vi "subParseForComponents.vi"(8 "error in (no error)":errorcluster, 9 "Parent layer":string, 10 "Parent component":string, 11 "Refnum in":refnum<k20>) -> (0 "error out":errorcluster, 1 "Rules":T1(array[cluster]), 3 "Refnum out":refnum<k20>)   [LabVIEW 2020, in "DefaultExtensions.lvlib" / "CDefaultRuleFileParser.lvclass"]
uses:
  CDefaultRuleFileParser.lvclass
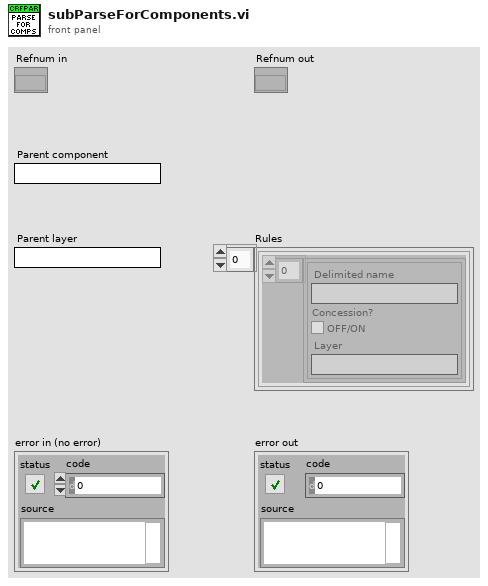
[diagram p1: front panel]
types:
  T1 = cluster{cluster{"Delimited name":string, "Concession?":bool, "Layer":string}[]}[]
  T2 = cluster{"Delimited name":string, "Concession?":bool, "Layer":string}
  T3 = cluster{"Delimited name":string, "Concession?":bool, "Layer":string}[]
  T4 = cluster{cluster{"Delimited name":string, "Concession?":bool, "Layer":string}[]}
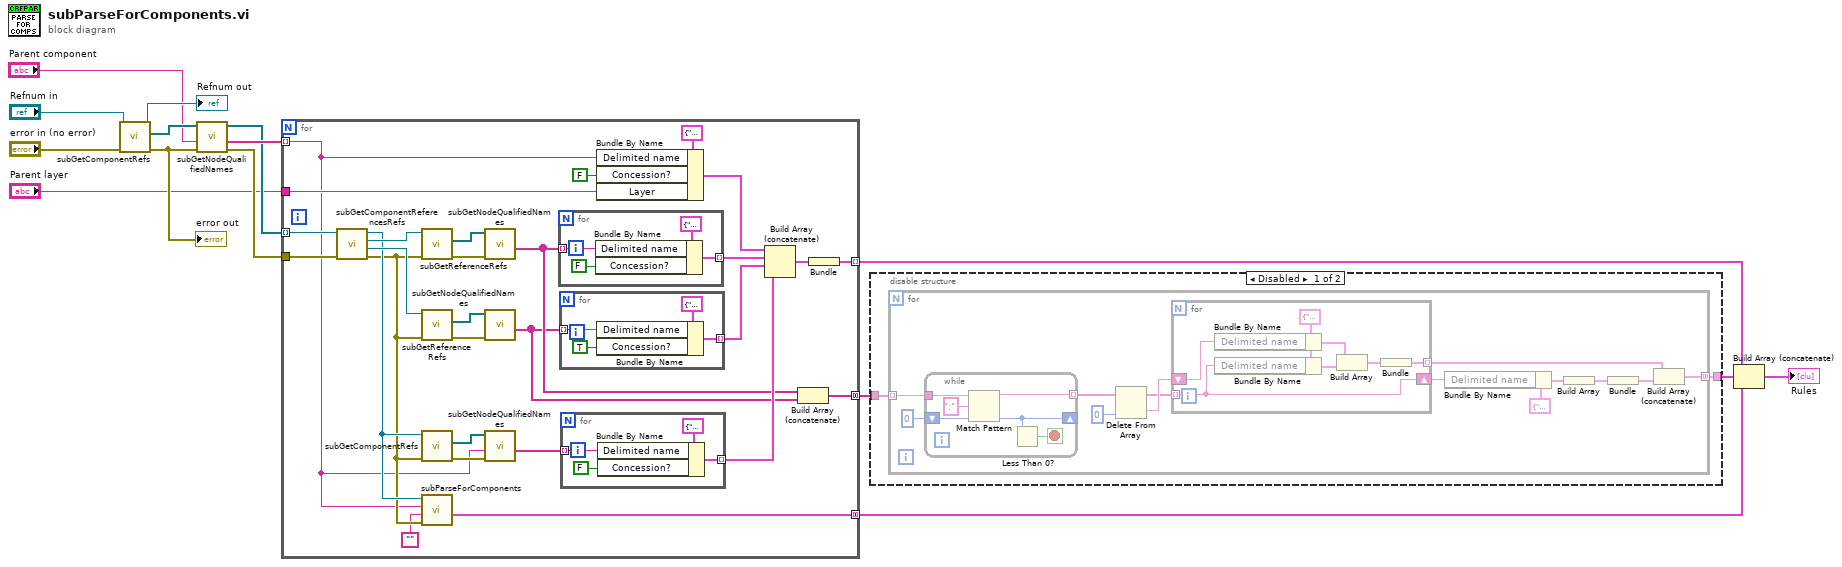
[diagram p0: block diagram]
diagram:
  n1 = call "subGetComponentRefs.vi"("error in (no error)"="error in (no error)", "Refnum in"="Refnum in") -> ("error out"=w15:errorcluster, "node result array"=w13:refnum<k20>[], "Refnum out"=→"Refnum out":refnum<k20>)  [unwired: 7 in]
  "error out" <- w15
  n2 = call "subGetNodeQualifiedNames.vi"("error in (no error)"=w15, "Parent node"="Parent component", "node[] in"=w13) -> ("error out"=w10:errorcluster, "node name[]"=w11:string[], "node[]"=w9:refnum<k20>[])  [unwired: 6 in]
  n3 = for {
    tunnel: w11 -> [w20] mode=indexing
    tunnel: [w34] -> w7 mode=indexing
    tunnel: w10 -> [w33]
    tunnel: w9 -> [w32] mode=indexing
    tunnel: "Parent layer" -> [w23]
    tunnel: [w28] -> w5 mode=concatenating
    tunnel: [w16] -> w1 mode=concatenating
    n4 = call "subGetComponentReferencesRefs.vi"("error in (no error)"=w33, "Refnum in"=w32) -> ("error out"=w24:errorcluster, "Concession Node Ref out"=w42:refnum<k20>, "Allow Node Ref out"=w43:refnum<k20>, "Refnum out"=w25:refnum<k20>)  [unwired: 6 in]
    n5 = call "subGetReferenceRefs.vi"("error in (no error)"=w24, "Refnum in"=w43) -> ("error out"=w40:errorcluster, "node result array"=w41:refnum<k20>[])  [unwired: 7 in, 1 out]
    n6 = call "subGetReferenceRefs.vi"("error in (no error)"=w24, "Refnum in"=w42) -> ("error out"=w38:errorcluster, "node result array"=w39:refnum<k20>[])  [unwired: 7 in, 1 out]
    n7 = call "subGetComponentRefs.vi"("error in (no error)"=w24, "Refnum in"=w25) -> ("error out"=w27:errorcluster, "node result array"=w26:refnum<k20>[])  [unwired: 7 in, 1 out]
    n8 = call "subParseForComponents.vi"("error in (no error)"=w24, "Parent layer"="", "Parent component"=w20, "Refnum in"=w25) -> ("Rules"=w28:T1)  [unwired: 5 in, 2 out]
    n9 = call "subGetNodeQualifiedNames.vi"("error in (no error)"=w40, "node[] in"=w41) -> ("node name[]"=w18:string[])  [unwired: 7 in, 2 out]
    n10 = call "subGetNodeQualifiedNames.vi"("error in (no error)"=w38, "node[] in"=w39) -> ("node name[]"=w17:string[])  [unwired: 7 in, 2 out]
    n11 = call "subGetNodeQualifiedNames.vi"("error in (no error)"=w27, "Parent node"=w20, "node[] in"=w26) -> ("node name[]"=w22:string[])  [unwired: 6 in, 2 out]
    n12 = for {
      tunnel: w18 -> [w54] mode=indexing
      tunnel: [w53] -> w37 mode=indexing
      n13 = Bundle By Name(cluster=T2 {"Delimited name"="", "Concession?"=FALSE, "Layer"=""} ("Cluster"), "Delimited name"=w54, "Concession?"=FALSE) -> (w53:T2)
    }
    n14 = for {
      tunnel: w17 -> [w50] mode=indexing
      tunnel: [w49] -> w36 mode=indexing
      n15 = Bundle By Name(cluster=T2 {"Delimited name"="", "Concession?"=FALSE, "Layer"=""} ("Cluster"), "Delimited name"=w50, "Concession?"=TRUE) -> (w49:T2)
    }
    n16 = for {
      tunnel: w22 -> [w46] mode=indexing
      tunnel: [w45] -> w21 mode=indexing
      n17 = Bundle By Name(cluster=T2 {"Delimited name"="", "Concession?"=FALSE, "Layer"=""} ("Cluster"), "Delimited name"=w46, "Concession?"=FALSE) -> (w45:T2)
    }
    n18 = Bundle By Name(cluster=T2 {"Delimited name"="", "Concession?"=FALSE, "Layer"=""} ("Cluster"), "Delimited name"=w20, "Concession?"=FALSE, "Layer"=w23) -> (w29:T2)
    n19 = Build Array (concatenate)(w29, w37, w36, w21) -> (w35:T3)
    n20 = Build Array (concatenate)(w18, w17) -> (w16:string[])
    n21 = Bundle(w35) -> (w34:T4)  [unwired: 1 in]
  }
  n22 = disable-structure shown="Disabled" {
    disable-tunnel: [w57 _] -> w2
    disable-tunnel: w1 -> [w56 _]
    frame Disabled {
      n23 = for {
        tunnel: w56 -> [w69] mode=indexing
        tunnel: [w58] -> w57 mode=concatenating
        n24 = while {
          tunnel: w69 -> [w83]
          shift-right: [w81] -> _
          shift-left: 0 ("offset past match") -> [w80]
          tunnel: [w78] -> w65 mode=indexing
          stop <- w79 stop-if-true
          n25 = Match Pattern(string=w83, regular expression=":" ("delimiter (Tab)"), offset (0)=w80) -> (before substring=w78:string, offset past match=w81:i32)  [unwired: 2 out]
          n26 = Less Than 0?(x=w81) -> (x < 0?=w79:bool)
        }
        n27 = Delete From Array(array=w65, index=0) -> (deleted portion=w67:string, array with subset deleted=w66:string[])  [unwired: 1 in]
        n28 = for {
          shift-right: [w73] -> w63
          shift-left: w67 -> [w75]
          tunnel: w66 -> [w73] mode=indexing
          tunnel: [w76] -> w60 mode=indexing
          w74 = T2 {"Delimited name"="", "Concession?"=FALSE, "Layer"=""} ("Cluster")
          n29 = Bundle By Name(cluster=w74, "Delimited name"=w75) -> (w72:T2)
          n30 = Bundle By Name(cluster=w74, "Delimited name"=w73) -> (w71:T2)
          n31 = Build Array(w72, w71) -> (w77:T3)
          n32 = Bundle(w77) -> (w76:T4)  [unwired: 1 in]
        }
        n33 = Bundle By Name(cluster=T2 {"Delimited name"="", "Concession?"=FALSE, "Layer"=""} ("Cluster"), "Delimited name"=w63) -> (w61:T2)
        n34 = Build Array(w61) -> (w62:T3)
        n35 = Bundle(w62) -> (w59:T4)  [unwired: 1 in]
        n36 = Build Array (concatenate)(w60, w59) -> (w58:T1)
      }
    }
    frame Enabled {
    }
  }
  n37 = Build Array (concatenate)(w7, w2, w5) -> (→"Rules":T1)
